vi "MC shot collector tester.vi"() -> ()   [LabVIEW 2020]
uses:
  Shared/MySQL/Preset Query Enum.ctl
panel:
  out "timeout":bool
  out "device times out":cluster{"Device":string, "time":u32}[](array[cluster])
  out "All data out":string[][](array[string])
  in  "Device/Devicetype name\n/Plotter.id/#":string
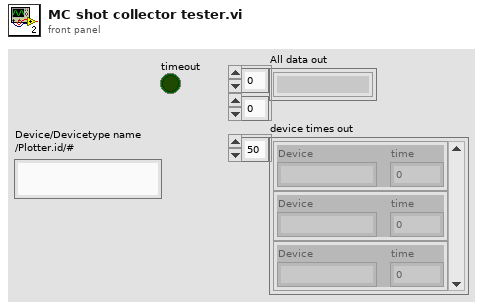
[diagram p1: front panel]
types:
  T1 = typedef "Preset Query Enum.ctl" = enum16{"Get Locations", "Get all IPs and MACs", "Get classes", "Get expt variables to set at scanstart for particular device", "Get expt devices and variables with start values", "Get expt devices and variables (with data to get)", "Get expt devices with data to get", "Get Expt devices and GUIs", "Get all devices basic properties", "Get Virtual Devices Core Info", "Get Expt names", "Get experiment basic properties", "Get experiment alarm variables", "Get MC Ports", "Get device network comm port", "Get devicetype lvclass path", "Get basic device properties", "Get Init Order", "Get all setable variables of a device", "Get device variable aliases", "Get force values of all settable variables", "Get all variables of a devicetype", "Get all variables of a device", "Get plotter details", "Get Saved Scans", "Get Scan Info", "GetGeneralGUIs", "Get expt for plotter", "Get plotter IDs from expt", "Get all devices", "Get all Virtual Devices", "Get all aliases", "Get variable and device info for Virtual Device", "GetItemLocatorIP", "Get IPs for GUIs", "Get DeviceType from Device", "GetLocalPortRange", "GetDevicePresetVariables", "Get Device Configuration", "GetAllPresetNames", "GetAllConfigurationNames", "GetPresetDeviceNames", "GetDeviceAliases", "GetDevicesOfClass"}
  T2 = typedef "TCP subscription info cluster.ctl" = cluster{"Device":string, "Variables":string[]}[]
  T3 = typedef "tcp_new_data_event.ctl" = refnum<user-event>
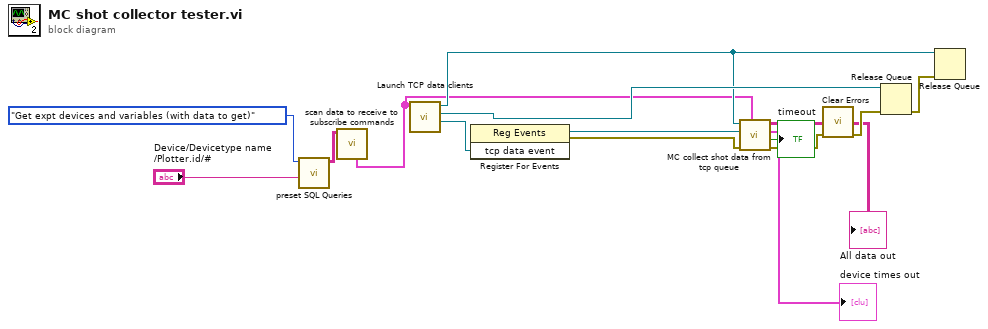
[diagram p0: block diagram]
diagram:
  n1 = call "preset SQL Queries.vi"("Expt name / MCIP/ Variable/Preset Name"="Device/Devicetype name\n/Plotter.id/#", "Preset Query"=Preset_Query_Enum."Get expt devices and variables (with data to get)") -> ("data"=w11:string[][])  [unwired: 7 in, 2 out]
  n2 = call "scan data to receive to subscribe commands.vi"("ScanData to receive"=w11) -> ("TCP subscriptions info"=w4:T2)  [unwired: 7 in, 3 out]
  n3 = call "Launch TCP data clients.vi"("TCP subscriptions info"=w4) -> ("tcp data event"=w14:T3, "StopQueue"=w15:refnum<queue>, "DataQueue"=w7:refnum<queue>)  [unwired: 8 in]
  n4 = register-events(w14) -> (reference out=w6:refnum<event-registration>, error out=w5:errorcluster)  [unwired: 2 in]
  n5 = call "MC collect shot data from tcp queue.vi"("TCP subscriptions info"=w4, "error in (no error)"=w5, "TCP data Event Registration Refnum"=w6, "TCPshotDataQueue"=w7) -> ("error out"=w10:errorcluster, "timeout"=→"timeout":bool, "device times out"=→"device times out":cluster{"Device":string, "time":u32}[], "All data out"=→"All data out":string[][])  [unwired: 4 in]
  n6 = call <vilib>:"Clear Errors.vi"("error in (no error)"=w10) -> ("error out"=w9:errorcluster)  [unwired: 5 in, 1 out]
  n7 = Release Queue(queue=w15, error in (no error)=w9) -> (error out=w8:errorcluster)  [unwired: 1 in, 2 out]
  n8 = Release Queue(queue=w7, error in (no error)=w8) -> ()  [unwired: 1 in, 3 out]
